vi "get channels.vi"(11 "fixed channel configuration in":refnum<class "fixed channel configuration.lvclass">) -> (2 "channels":refnum<class "TBM channel.lvclass">[](array[class]), 3 "fixed channel configuration out":refnum<class "fixed channel configuration.lvclass">)   [LabVIEW 2013, in "fixed channel configuration.lvclass"]
uses:
  fixed channel configuration.lvclass
  <vilib>/NI/Tag Bus Module Framework/channel/TBM channel.lvclass
  fixed channel configuration.lvclass/fixed channel configuration.ctl
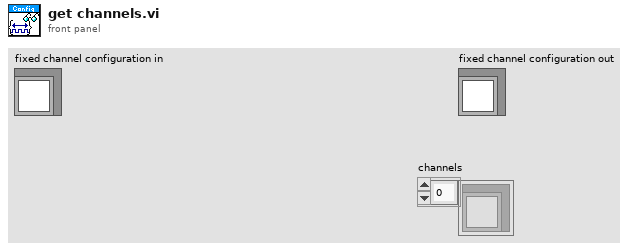
[diagram p1: front panel]
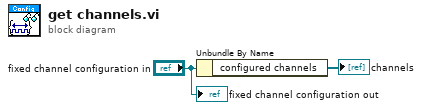
[diagram p0: block diagram]
diagram:
  n1 = Unbundle By Name("fixed channel configuration in") -> ("configured channels"=→"channels":refnum<class "TBM channel.lvclass">[])
  "fixed channel configuration out" <- "fixed channel configuration in"
